vi "solar_write SOLARUIUnhide.vi"(8 "error in (no error)":errorcluster, 10 "Target":string, 11 "solar in":refnum<class "solar.lvclass">) -> (0 "error out":errorcluster, 3 "solar out":refnum<class "solar.lvclass">)   [LabVIEW 2018, in "solar.lvclass"]
doc: "This shows a target in the Target List."
uses:
  solar.lvclass
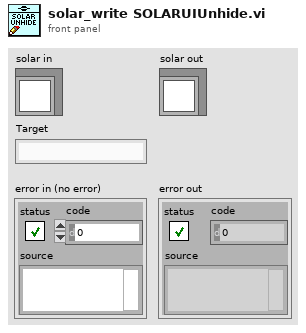
[diagram p1: front panel]
types:
  T1 = typedef "solar_ctl SOLAR Refnum.ctl" = refnum<k1>
  T2 = typedef "solar_ctl SOLAR Global.ctl" = cluster{"Targets":T3[], "AppDir":path, "solar.ini":path, "ConfigsDir":path, "CosmosDir":path, "LogsDir":path, "ExePath":path, "ExeVersion":string, "PartNum":string, "AppSetup":string, "Title":string, "Main.ini":path, "Temp.ini":path, "vSOLAR":string, "Splash.png":string, "SplashWait":i32, "SOLARUE":refnum<user-event>, "VoyagerRefnum":T4, "QTimerRefnum":T5}
  T3 = typedef "solar_ctl Target Global.ctl" = cluster{"Target":string, "Q":refnum<queue>, "UE":refnum<user-event>, "VI":refnum<vi>, "Menu":refnum<k9>, "Data":refnum<data-value>, "Attributes":variant}
  T4 = typedef "solar_voy_ctl Voyager Refnum.ctl" = refnum<k1>
  T5 = typedef "solar_qtimer_ctl Refnum.ctl" = refnum<k1>
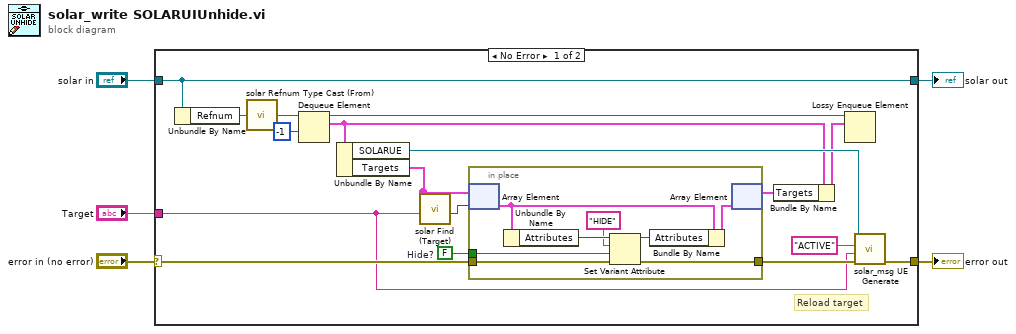
[diagram p0: block diagram]
diagram:
  n1 = case shown="No Error" "error in (no error)" {
    selector: "error in (no error)" -> [w16 w32]
    tunnel: "solar in" -> [w22 w31]
    tunnel: [w19 w32] -> w1
    tunnel: [w22 w31] -> w2
    tunnel: "Target" -> [w6 _]
    frame No Error {
      w7 = FALSE  # Hide?
      # "Reload target"
      n2 = Unbundle By Name(w22) -> ("Refnum"=w14:T1)
      n3 = call "solar Refnum Type Cast (From).vi"("Refnum"=w14) -> ("SOLAR"=w13:refnum<queue>)
      n4 = Dequeue Element(queue=w13, timeout in ms (-1)=-1) -> (queue out=w12:refnum<queue>, element=w11:T2)  [unwired: 1 in, 2 out]
      n5 = Unbundle By Name(w11) -> ("SOLARUE"=w20:refnum<user-event>, "Targets"=w18:T3[])
      n6 = call "solar Find (Target).vi"("Target"=w6, "Targets"=w18) -> ("Target Index"=w17:i32)  [unwired: 8 in, 1 out]
      n7 = in-place {
        in-place-border: w16 -> [w25]
        in-place-border: [w24] -> w15
        in-place-border: w7 -> [w23]
        n8 = in-place-array #1(w18, w17) -> (w30:T3)
        n9 = Unbundle By Name(w30) -> ("Attributes"=w28:variant)
        n10 = Set Variant Attribute(Variant=w28, name="HIDE", value=w23, error in=w25) -> (Variant out=w26:variant, error out=w24:errorcluster)  [unwired: 1 out]
        n11 = Bundle By Name(cluster=w30, "Attributes"=w26) -> (w29:T3)
        n12 = in-place-array #1(w29) -> (w10:T3[])  [unwired: 1 out]
      }
      n13 = Bundle By Name(cluster=w11, "Targets"=w10) -> (w9:T2)
      n14 = Lossy Enqueue Element(queue=w12, element=w9) -> ()  [unwired: 1 in, 4 out]
      n15 = call "solar_msg UE Generate.vi"("error in (no error)"=w15, "CMD_DATA (Last)"=w6, "CMD (Last)"="ACTIVE" ("Packet"), "UserEvent in"=w20) -> ("error out"=w19:errorcluster)  [unwired: 6 in, 1 out]
    }
    frame Error {
    }
  }
  "error out" <- w1
  "solar out" <- w2
